vi "Append Data.vi"(8 "error in (no error)":errorcluster, 9 "Data":variant, 10 "ParamTags":T1, 11 "Waveforms Common Methods in":refnum<class "Waveforms Common Methods.lvclass">) -> (0 "error out":errorcluster, 3 "Waveforms Common Methods out":refnum<class "Waveforms Common Methods.lvclass">)   [LabVIEW 2021, in "Rigol DG822 UI.lvlib" / "Waveforms Common Methods.lvclass"]
uses:
  Waveforms Common Methods.lvclass
  lib/controls.llb/WaveformParamTags.ctl
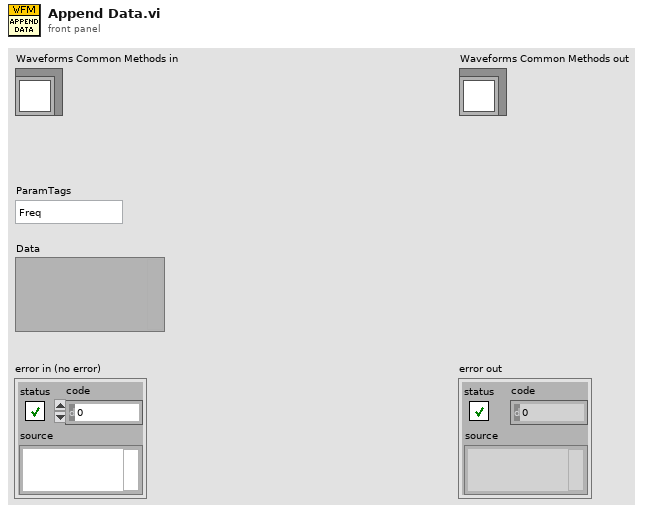
[diagram p1: front panel]
types:
  T1 = typedef "WaveformParamTags.ctl" = enum16{"Freq", "Period", "Ampl", "HighL", "Offset", "LowL", "Phase", "Duty", "Width", "RisEdge", "FallEdge"}
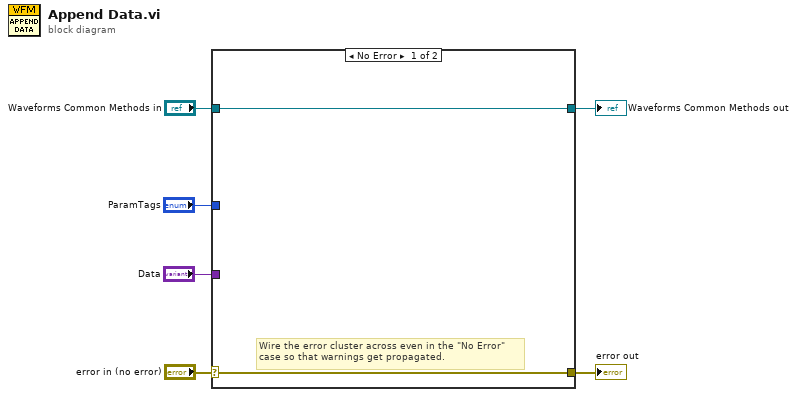
[diagram p0: block diagram]
diagram:
  n1 = case shown="No Error" "error in (no error)" {
    selector: "error in (no error)" -> [w7 w10]
    tunnel: [w7 w10] -> w5
    tunnel: [w8 w9] -> w3
    tunnel: "Waveforms Common Methods in" -> [w8 w9]
    tunnel: "Data" -> [_ _]
    tunnel: "ParamTags" -> [_ _]
    frame No Error {
      # "Wire the error cluster across even in the \"No Error\"\ncase so that warnings get propagated."
    }
    frame Error {
    }
  }
  "error out" <- w5
  "Waveforms Common Methods out" <- w3
